vi "_backward.vi"(8 "i":errorcluster, 11 "In":refnum<class "Value.lvclass">) -> (0 "error out":errorcluster, 3 "Out":refnum<class "Value.lvclass">)   [LabVIEW 2023, in "LabGRAD.lvlib" / "Value.lvclass"]
uses:
  Value.lvclass
  Value.lvclass/Value.ctl
  get set ini.ctl
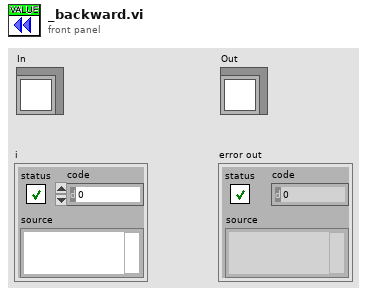
[diagram p1: front panel]
types:
  T1 = typedef "LabGRAD.lvlib/Value.lvclass/get set ini.ctl" = enum16{"get", "set", "ini"}
  T2 = typedef "LabGRAD.lvlib/Value.lvclass/operation.ctl" = enum16{"nop", "add", "subtract", "power", "multiply", "divide", "tanh"}
  T3 = typedef "UiObjects.lvlib/UiObjects.lvclass/numeric value control.ctl" = dbl
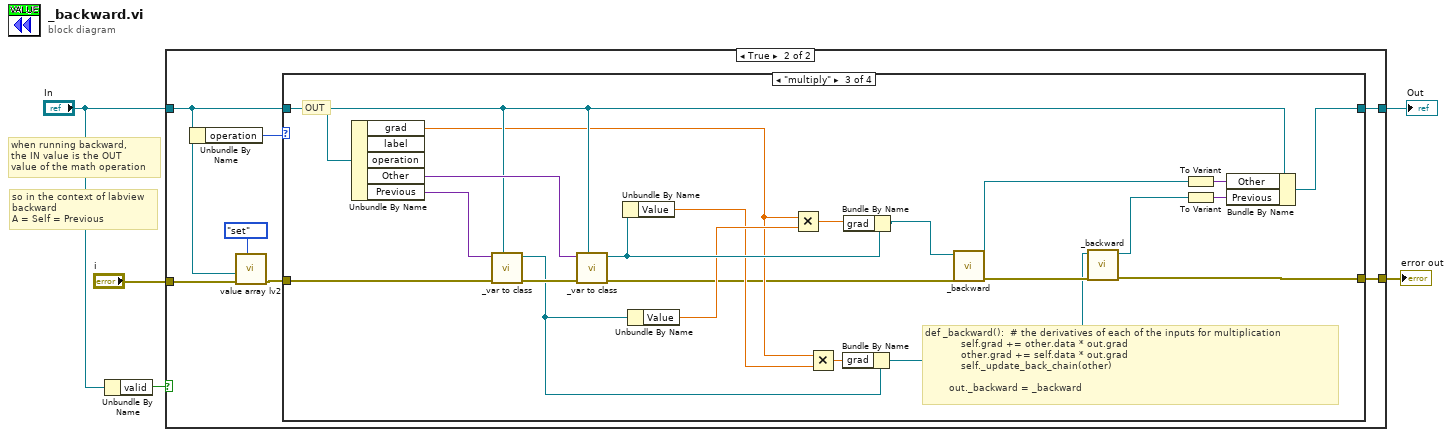
[diagram p0: block diagram]
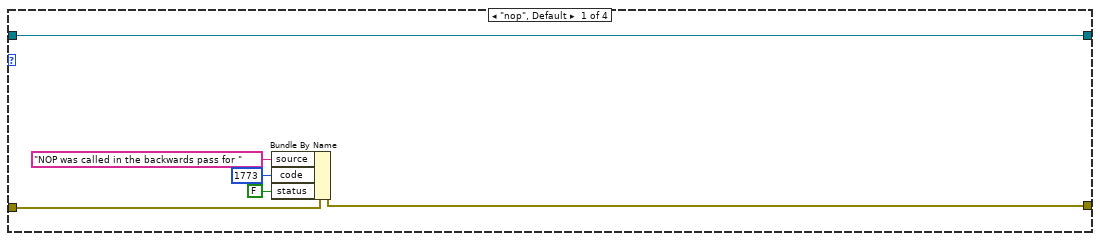
[diagram p3: hidden frame]
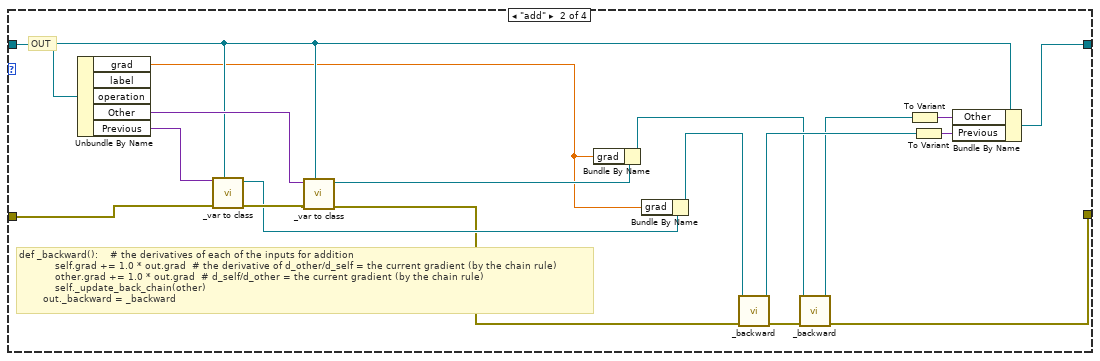
[diagram p4: hidden frame]
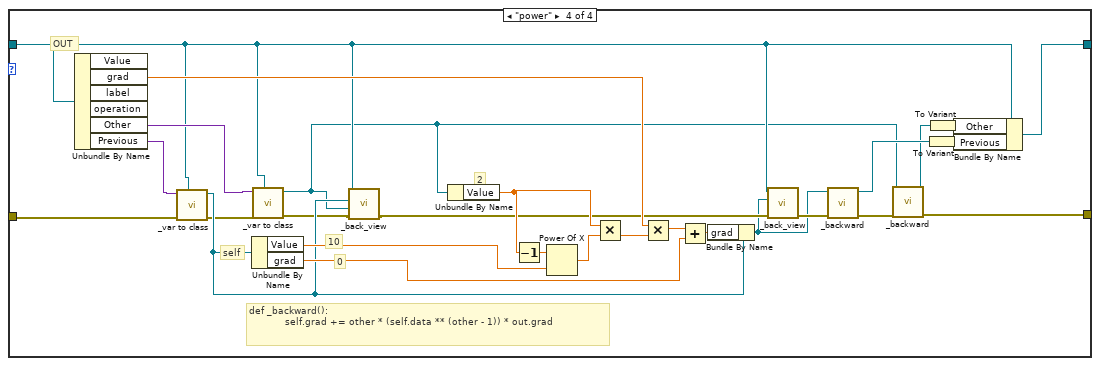
[diagram p5: hidden frame]
diagram:
  # "so in the context of labview\nbackward\nA = Self = Previous"
  # "when running backward, \nthe IN value is the OUT\nvalue of the math operation"
  n1 = Unbundle By Name("In") -> ("valid"=w1:bool)
  n2 = case shown="True" w1 {
    tunnel: [w6 w12] -> w5
    tunnel: [w7 w14] -> w4
    tunnel: "In" -> [w7 w8]
    tunnel: "i" -> [w6 w11]
    frame False {
    }
    frame True {
      n3 = Unbundle By Name(w8) -> ("operation"=w13:T2)
      n4 = call "value array lv2.vi"("Enum"=get_set_ini."set", "i"=w11, "Value in"=w8) -> ("out"=w10:errorcluster)  [unwired: 5 in, 2 out]
      n5 = case shown="\"multiply\"" w13 {
        tunnel: w8 -> [w20 w34 w55 w65]
        tunnel: [w20 w38 w60 w87] -> w14
        tunnel: w10 -> [w19 w37 w58 w63]
        tunnel: [w18 w25 w39 w69] -> w12
        frame "nop", Default {
          n6 = Bundle By Name(cluster=w19, "source"="NOP was called in the backwards pass for ", "code"=1773, "status"=FALSE) -> (w18:errorcluster)
        }
        frame "add" {
          # "def _backward():    # the derivatives of each of the inputs for addition\n            self.grad += 1.0 * out.grad  # the derivative of d_other/d_self = the current gradient (by the chain rule)\n            other.grad += 1.0 * out.grad  # d_self/d_other = the current gradient (by the chain rule)\n            self._update_back_chain(other)\n        out._backward = _backward"
          # "OUT"
          n7 = Unbundle By Name(w34) -> ("grad"=w30:T3, "Other"=w35:variant, "Previous"=w36:variant)  [unwired: 2 out]
          n8 = call "_var to class.vi"("In"=w34, "error in"=w37, "variant"=w36) -> ("error out"=w33:errorcluster, "Out"=w31:refnum<class "Value.lvclass">)  [unwired: 6 in, 1 out]
          n9 = call "_var to class.vi"("In"=w34, "error in"=w33, "variant"=w35) -> ("error out"=w27:errorcluster, "Out"=w32:refnum<class "Value.lvclass">)  [unwired: 6 in, 1 out]
          n10 = Bundle By Name(cluster=w32, "grad"=w30) -> (w22:refnum<class "Value.lvclass">)
          n11 = Bundle By Name(cluster=w31, "grad"=w30) -> (w24:refnum<class "Value.lvclass">)
          n12 = call "_backward.vi"("i"=w27, "In"=w24) -> ("error out"=w26:errorcluster, "Out"=w23:refnum<class "Value.lvclass">)  [unwired: 8 in]
          n13 = call "_backward.vi"("i"=w26, "In"=w22) -> ("error out"=w25:errorcluster, "Out"=w21:refnum<class "Value.lvclass">)  [unwired: 8 in]
          n14 = To Variant(anything=w21) -> (Variant=w29:variant)
          n15 = To Variant(anything=w23) -> (Variant=w28:variant)
          n16 = Bundle By Name(cluster=w34, "Other"=w29, "Previous"=w28) -> (w38:refnum<class "Value.lvclass">)
        }
        frame "multiply" {
          # "def _backward():  # the derivatives of each of the inputs for multiplication\n            self.grad += other.data * out.grad\n            other.grad += self.data * out.grad\n            self._update_back_chain(other)\n\n        out._backward = _backward"
          # "OUT"
          n17 = Unbundle By Name(w55) -> ("grad"=w50:T3, "Other"=w57:variant, "Previous"=w59:variant)  [unwired: 2 out]
          n18 = call "_var to class.vi"("In"=w55, "error in"=w58, "variant"=w59) -> ("error out"=w56:errorcluster, "Out"=w53:refnum<class "Value.lvclass">)  [unwired: 6 in, 1 out]
          n19 = call "_var to class.vi"("In"=w55, "error in"=w56, "variant"=w57) -> ("error out"=w46:errorcluster, "Out"=w54:refnum<class "Value.lvclass">)  [unwired: 6 in, 1 out]
          n20 = Unbundle By Name(w54) -> ("Value"=w49:T3)
          n21 = Unbundle By Name(w53) -> ("Value"=w52:T3)
          n22 = Multiply(x=w50, y=w52) -> (x*y=w51:T3)
          n23 = Multiply(x=w50, y=w49) -> (x*y=w48:T3)
          n24 = Bundle By Name(cluster=w53, "grad"=w48) -> (w44:refnum<class "Value.lvclass">)
          n25 = Bundle By Name(cluster=w54, "grad"=w51) -> (w47:refnum<class "Value.lvclass">)
          n26 = call "_backward.vi"("i"=w46, "In"=w47) -> ("error out"=w45:errorcluster, "Out"=w43:refnum<class "Value.lvclass">)  [unwired: 8 in]
          n27 = call "_backward.vi"("i"=w45, "In"=w44) -> ("error out"=w39:errorcluster, "Out"=w42:refnum<class "Value.lvclass">)  [unwired: 8 in]
          n28 = To Variant(anything=w43) -> (Variant=w41:variant)
          n29 = To Variant(anything=w42) -> (Variant=w40:variant)
          n30 = Bundle By Name(cluster=w55, "Other"=w41, "Previous"=w40) -> (w60:refnum<class "Value.lvclass">)
        }
        frame "power" {
          # "0"
          # "10"
          # "2"
          # "self"
          # "def _backward():\n            self.grad += other * (self.data ** (other - 1)) * out.grad"
          # "OUT"
          n31 = Unbundle By Name(w65) -> ("grad"=w86:T3, "Other"=w66:variant, "Previous"=w68:variant)  [unwired: 3 out]
          n32 = call "_var to class.vi"("In"=w65, "error in"=w63, "variant"=w68) -> ("error out"=w62:errorcluster, "Out"=w67:refnum<class "Value.lvclass">)  [unwired: 6 in, 1 out]
          n33 = Unbundle By Name(w67) -> ("Value"=w81:T3, "grad"=w84:T3)
          n34 = call "_var to class.vi"("In"=w65, "error in"=w62, "variant"=w66) -> ("error out"=w61:errorcluster, "Out"=w64:refnum<class "Value.lvclass">)  [unwired: 6 in, 1 out]
          n35 = call "_back_view.vi"("error in (no error)"=w61, "other"=w64, "prev"=w67, "IN"=w65) -> ("error out"=w75:errorcluster)  [unwired: 1 in, 6 out]
          n36 = Unbundle By Name(w64) -> ("Value"=w76:T3)
          n37 = Decrement(x=w76) -> (x-1=w79:T3)
          n38 = Power Of X(1:w81, 2:w79) -> (0:w80:T3)
          n39 = Multiply(x=w76, y=w80) -> (x*y=w77:T3)
          n40 = Multiply(x=w86, y=w77) -> (x*y=w78:T3)
          n41 = Add(x=w78, y=w84) -> (x+y=w83:T3)
          n42 = Bundle By Name(cluster=w67, "grad"=w83) -> (w72:refnum<class "Value.lvclass">)
          n43 = call "_back_view.vi"("error in (no error)"=w75, "prev"=w72, "IN"=w65) -> ("error out"=w74:errorcluster)  [unwired: 2 in, 6 out]
          n44 = call "_backward.vi"("i"=w74, "In"=w72) -> ("error out"=w73:errorcluster, "Out"=w71:refnum<class "Value.lvclass">)  [unwired: 8 in]
          n45 = call "_backward.vi"("i"=w73, "In"=w64) -> ("error out"=w69:errorcluster, "Out"=w70:refnum<class "Value.lvclass">)  [unwired: 8 in]
          n46 = To Variant(anything=w71) -> (Variant=w82:variant)
          n47 = To Variant(anything=w70) -> (Variant=w85:variant)
          n48 = Bundle By Name(cluster=w65, "Other"=w85, "Previous"=w82) -> (w87:refnum<class "Value.lvclass">)
        }
      }
    }
  }
  "error out" <- w5
  "Out" <- w4
